vi "Three part live.vi"() -> ()   [LabVIEW 2009]
uses:
  <vilib>/vision/Image Controls.llb/IMAQ Image.ctl
  <vilib>/Instr/_visa.llb/VISA Configure Serial Port (Instr).vi
  <vilib>/userDefined/High Color/IMAQdx.ctl
  <vilib>/Analysis/3filter.llb/Filter Passband Type.ctl
  <vilib>/Analysis/3filter.llb/Butterworth Filter (DBL).vi
  <vilib>/vision/NI_Vision_Development_Module.lvlib
  <vilib>/Analysis/NI_AALBase.lvlib
  <vilib>/vision/driver/NI_Vision_Acquisition_Software.lvlib
panel:
  in  "Orange Guitar":T1={"Global Rectangle"=[587, 282, 628, 378], "Contours"=[{"ID"=enum."External", "Type"=2, "Coordinates"=[627, 377, 587, 282]}]} {"Contours"."Type" items=["No Selection", "Point", "Line", "Rectangle", "Oval", "Polygon", "Freehand Region", "Annulus", "Unused2", "Unused3", "Broken Line", "Freehand Line", "Rotated Rectangle"]}
  in  "Yellow Guitar":T1={"Global Rectangle"=[546, 282, 563, 376], "Contours"=[{"ID"=enum."External", "Type"=2, "Coordinates"=[562, 375, 546, 282]}]} {"Contours"."Type" items=["No Selection", "Point", "Line", "Rectangle", "Oval", "Polygon", "Freehand Region", "Annulus", "Unused2", "Unused3", "Broken Line", "Freehand Line", "Rotated Rectangle"]}
  in  "Green Guitar":T1={"Global Rectangle"=[498, 284, 505, 376], "Contours"=[{"ID"=enum."External", "Type"=2, "Coordinates"=[498, 375, 504, 284]}]} {"Contours"."Type" items=["No Selection", "Point", "Line", "Rectangle", "Oval", "Polygon", "Freehand Region", "Annulus", "Unused2", "Unused3", "Broken Line", "Freehand Line", "Rotated Rectangle"]}
  in  "Blue Guitar":T1={"Global Rectangle"=[569, 290, 594, 372], "Contours"=[{"ID"=enum."External", "Type"=2, "Coordinates"=[593, 371, 569, 290]}]} {"Contours"."Type" items=["No Selection", "Point", "Line", "Rectangle", "Oval", "Polygon", "Freehand Region", "Annulus", "Unused2", "Unused3", "Broken Line", "Freehand Line", "Rotated Rectangle"]}
  in  "Red Guitar":T1={"Global Rectangle"=[526, 284, 530, 370], "Contours"=[{"ID"=enum."External", "Type"=2, "Coordinates"=[529, 369, 526, 284]}]} {"Contours"."Type" items=["No Selection", "Point", "Line", "Rectangle", "Oval", "Polygon", "Freehand Region", "Annulus", "Unused2", "Unused3", "Broken Line", "Freehand Line", "Rotated Rectangle"]}
  in  "sampling  9":dbl=1.0 format="%0.2f"
  in  "high 14":dbl=60.0 format="%0.2f"
  out "Blue Guitar":dbl[](graph)
  in  "low 3":dbl=0.12500000000000006 format="%0.4f"
  out "Yellow Guitar":dbl[](graph)
  out "Yellow Guitar LED":bool
  in  "sampling 12":dbl=1.0 format="%0.2f"
  in  "high 13":dbl=60.0 format="%0.2f"
  in  "low  12":dbl=0.12500000000000006 format="%0.4f"
  out "Yellow Guitar":T1={"Global Rectangle"=[243, 262, 261, 384], "Contours"=[{"ID"=enum."External", "Type"=2, "Coordinates"=[260, 383, 243, 262]}]} {"Contours"."Type" items=["No Selection", "Point", "Line", "Rectangle", "Oval", "Polygon", "Freehand Region", "Annulus", "Unused2", "Unused3", "Broken Line", "Freehand Line", "Rotated Rectangle"]}
  out "Blue Guitar":T1={"Global Rectangle"=[168, 264, 180, 378], "Contours"=[{"ID"=enum."External", "Type"=2, "Coordinates"=[168, 377, 179, 264]}]} {"Contours"."Type" items=["No Selection", "Point", "Line", "Rectangle", "Oval", "Polygon", "Freehand Region", "Annulus", "Unused2", "Unused3", "Broken Line", "Freehand Line", "Rotated Rectangle"]}
  out "Green Guitar":dbl[](graph)
  out "Green Guitar LED":bool
  in  "sampling 11":dbl=1.0 format="%0.2f"
  in  "high 12":dbl=60.0 format="%0.2f"
  in  "low  11":dbl=0.12500000000000006 format="%0.4f"
  out "Green Guitar":T1={"Global Rectangle"=[406, 309, 423, 383], "Contours"=[{"ID"=enum."External", "Type"=2, "Coordinates"=[422, 382, 406, 309]}]} {"Contours"."Type" items=["No Selection", "Point", "Line", "Rectangle", "Oval", "Polygon", "Freehand Region", "Annulus", "Unused2", "Unused3", "Broken Line", "Freehand Line", "Rotated Rectangle"]}
  out "Red Guitar":dbl[](graph)
  out "Red Guitar LED":bool
  in  "sampling 10":dbl=1.0 format="%0.2f"
  in  "high 11":dbl=60.0 format="%0.2f"
  in  "low  10":dbl=0.12500000000000006 format="%0.4f"
  out "Red Guitar":T1={"Global Rectangle"=[300, 297, 320, 380], "Contours"=[{"ID"=enum."External", "Type"=2, "Coordinates"=[300, 379, 319, 297]}]} {"Contours"."Type" items=["No Selection", "Point", "Line", "Rectangle", "Oval", "Polygon", "Freehand Region", "Annulus", "Unused2", "Unused3", "Broken Line", "Freehand Line", "Rotated Rectangle"]}
  out "Blue Guitar LED":bool
  out "Orange Guitar":dbl[](graph)
  out "Orange Guitar LED":bool
  in  "sampling 9":dbl=1.0 format="%0.2f"
  in  "high 10":dbl=60.0 format="%0.2f"
  in  "low  9":dbl=0.12500000000000006 format="%0.4f"
  out "Orange Guitar":T1={"Global Rectangle"=[300, 297, 320, 380], "Contours"=[{"ID"=enum."External", "Type"=2, "Coordinates"=[300, 379, 319, 297]}]} {"Contours"."Type" items=["No Selection", "Point", "Line", "Rectangle", "Oval", "Polygon", "Freehand Region", "Annulus", "Unused2", "Unused3", "Broken Line", "Freehand Line", "Rotated Rectangle"]}
  in  "Orange Bass":T1={"Global Rectangle"=[220, 296, 225, 371], "Contours"=[{"ID"=enum."External", "Type"=2, "Coordinates"=[224, 370, 220, 296]}]} {"Contours"."Type" items=["No Selection", "Point", "Line", "Rectangle", "Oval", "Polygon", "Freehand Region", "Annulus", "Unused2", "Unused3", "Broken Line", "Freehand Line", "Rotated Rectangle"]}
  out "Orange Bass":dbl[](graph)
  out "Orange Bass LED":bool
  in  "sampling 8":dbl=1.0 format="%0.2f"
  in  "high 9":dbl=60.0 format="%0.2f"
  in  "low  8":dbl=0.12500000000000006 format="%0.4f"
  out "Orange Bass":T1={"Global Rectangle"=[300, 297, 320, 380], "Contours"=[{"ID"=enum."External", "Type"=2, "Coordinates"=[300, 379, 319, 297]}]} {"Contours"."Type" items=["No Selection", "Point", "Line", "Rectangle", "Oval", "Polygon", "Freehand Region", "Annulus", "Unused2", "Unused3", "Broken Line", "Freehand Line", "Rotated Rectangle"]}
  in  "Green Bass":T1={"Global Rectangle"=[100, 292, 131, 371], "Contours"=[{"ID"=enum."External", "Type"=2, "Coordinates"=[100, 370, 130, 292]}]} {"Contours"."Type" items=["No Selection", "Point", "Line", "Rectangle", "Oval", "Polygon", "Freehand Region", "Annulus", "Unused2", "Unused3", "Broken Line", "Freehand Line", "Rotated Rectangle"]}
  in  "Blue Bass":T1={"Global Rectangle"=[193, 293, 199, 374], "Contours"=[{"ID"=enum."External", "Type"=2, "Coordinates"=[193, 373, 198, 293]}]} {"Contours"."Type" items=["No Selection", "Point", "Line", "Rectangle", "Oval", "Polygon", "Freehand Region", "Annulus", "Unused2", "Unused3", "Broken Line", "Freehand Line", "Rotated Rectangle"]}
  in  "Red Bass":T1={"Global Rectangle"=[129, 294, 154, 376], "Contours"=[{"ID"=enum."External", "Type"=2, "Coordinates"=[129, 375, 153, 294]}]} {"Contours"."Type" items=["No Selection", "Point", "Line", "Rectangle", "Oval", "Polygon", "Freehand Region", "Annulus", "Unused2", "Unused3", "Broken Line", "Freehand Line", "Rotated Rectangle"]}
  in  "Yellow Bass":T1={"Global Rectangle"=[160, 295, 175, 378], "Contours"=[{"ID"=enum."External", "Type"=2, "Coordinates"=[160, 377, 174, 295]}]} {"Contours"."Type" items=["No Selection", "Point", "Line", "Rectangle", "Oval", "Polygon", "Freehand Region", "Annulus", "Unused2", "Unused3", "Broken Line", "Freehand Line", "Rotated Rectangle"]}
  in  "sampling  8":dbl=1.0 format="%0.2f"
  in  "high 8":dbl=60.0 format="%0.2f"
  out "Blue Bass":dbl[](graph)
  in  "low 2":dbl=0.12500000000000006 format="%0.4f"
  out "Yellow Bass":dbl[](graph)
  out "Yellow Bass LED":bool
  in  "sampling 7":dbl=1.0 format="%0.2f"
  in  "high 7":dbl=60.0 format="%0.2f"
  in  "low  7":dbl=0.12500000000000006 format="%0.4f"
  out "Yellow Bass":T1={"Global Rectangle"=[243, 262, 261, 384], "Contours"=[{"ID"=enum."External", "Type"=2, "Coordinates"=[260, 383, 243, 262]}]} {"Contours"."Type" items=["No Selection", "Point", "Line", "Rectangle", "Oval", "Polygon", "Freehand Region", "Annulus", "Unused2", "Unused3", "Broken Line", "Freehand Line", "Rotated Rectangle"]}
  out "Blue Bass":T1={"Global Rectangle"=[168, 264, 180, 378], "Contours"=[{"ID"=enum."External", "Type"=2, "Coordinates"=[168, 377, 179, 264]}]} {"Contours"."Type" items=["No Selection", "Point", "Line", "Rectangle", "Oval", "Polygon", "Freehand Region", "Annulus", "Unused2", "Unused3", "Broken Line", "Freehand Line", "Rotated Rectangle"]}
  out "Green Bass":dbl[](graph)
  out "Green Bass LED":bool
  in  "sampling 6":dbl=1.0 format="%0.2f"
  in  "high 6":dbl=60.0 format="%0.2f"
  in  "low  6":dbl=0.12500000000000006 format="%0.4f"
  out "Green Bass":T1={"Global Rectangle"=[406, 309, 423, 383], "Contours"=[{"ID"=enum."External", "Type"=2, "Coordinates"=[422, 382, 406, 309]}]} {"Contours"."Type" items=["No Selection", "Point", "Line", "Rectangle", "Oval", "Polygon", "Freehand Region", "Annulus", "Unused2", "Unused3", "Broken Line", "Freehand Line", "Rotated Rectangle"]}
  out "Red Bass":dbl[](graph)
  out "Red Bass LED":bool
  in  "sampling 5":dbl=1.0 format="%0.2f"
  in  "high 5":dbl=60.0 format="%0.2f"
  in  "low  5":dbl=0.12500000000000006 format="%0.4f"
  out "Red Bass":T1={"Global Rectangle"=[300, 297, 320, 380], "Contours"=[{"ID"=enum."External", "Type"=2, "Coordinates"=[300, 379, 319, 297]}]} {"Contours"."Type" items=["No Selection", "Point", "Line", "Rectangle", "Oval", "Polygon", "Freehand Region", "Annulus", "Unused2", "Unused3", "Broken Line", "Freehand Line", "Rotated Rectangle"]}
  out "Blue Bass LED":bool
  in  "Mask":T1 {"Contours"."Type" items=["No Selection", "Point", "Line", "Rectangle", "Oval", "Polygon", "Freehand Region", "Annulus", "Unused2", "Unused3", "Broken Line", "Freehand Line", "Rotated Rectangle"]}
  out "Image 2":T2(plugin-control)
  out "Red Line":T1={"Global Rectangle"=[300, 297, 320, 380], "Contours"=[{"ID"=enum."External", "Type"=2, "Coordinates"=[300, 379, 319, 297]}]} {"Contours"."Type" items=["No Selection", "Point", "Line", "Rectangle", "Oval", "Polygon", "Freehand Region", "Annulus", "Unused2", "Unused3", "Broken Line", "Freehand Line", "Rotated Rectangle"]}
  in  "Red Line":T1={"Global Rectangle"=[300, 297, 320, 380], "Contours"=[{"ID"=enum."External", "Type"=2, "Coordinates"=[300, 379, 319, 297]}]} {"Contours"."Type" items=["No Selection", "Point", "Line", "Rectangle", "Oval", "Polygon", "Freehand Region", "Annulus", "Unused2", "Unused3", "Broken Line", "Freehand Line", "Rotated Rectangle"]}
  out "Waveform Red":dbl[](graph)
  out "LED Red":bool
  in  "sampling 4":dbl=1.0 format="%0.2f"
  in  "high 4":dbl=60.0 format="%0.2f"
  in  "low  4":dbl=0.12500000000000006 format="%0.4f"
  out "Green Line":T1={"Global Rectangle"=[406, 309, 423, 383], "Contours"=[{"ID"=enum."External", "Type"=2, "Coordinates"=[422, 382, 406, 309]}]} {"Contours"."Type" items=["No Selection", "Point", "Line", "Rectangle", "Oval", "Polygon", "Freehand Region", "Annulus", "Unused2", "Unused3", "Broken Line", "Freehand Line", "Rotated Rectangle"]}
  in  "Blue Line":T1={"Global Rectangle"=[374, 278, 383, 377], "Contours"=[{"ID"=enum."External", "Type"=2, "Coordinates"=[382, 376, 374, 278]}]} {"Contours"."Type" items=["No Selection", "Point", "Line", "Rectangle", "Oval", "Polygon", "Freehand Region", "Annulus", "Unused2", "Unused3", "Broken Line", "Freehand Line", "Rotated Rectangle"]}
  in  "Green Line":T1={"Global Rectangle"=[406, 309, 423, 383], "Contours"=[{"ID"=enum."External", "Type"=2, "Coordinates"=[422, 382, 406, 309]}]} {"Contours"."Type" items=["No Selection", "Point", "Line", "Rectangle", "Oval", "Polygon", "Freehand Region", "Annulus", "Unused2", "Unused3", "Broken Line", "Freehand Line", "Rotated Rectangle"]}
  in  "low  3":dbl=0.12500000000000006 format="%0.4f"
  out "Waveform Green":dbl[](graph)
  out "LED Green":bool
  in  "sampling 3":dbl=1.0 format="%0.2f"
  in  "high 3":dbl=60.0 format="%0.2f"
  in  "Yellow Line":T1={"Global Rectangle"=[342, 292, 349, 377], "Contours"=[{"ID"=enum."External", "Type"=2, "Coordinates"=[342, 376, 348, 292]}]} {"Contours"."Type" items=["No Selection", "Point", "Line", "Rectangle", "Oval", "Polygon", "Freehand Region", "Annulus", "Unused2", "Unused3", "Broken Line", "Freehand Line", "Rotated Rectangle"]}
  out "Blue Line":T1={"Global Rectangle"=[168, 264, 180, 378], "Contours"=[{"ID"=enum."External", "Type"=2, "Coordinates"=[168, 377, 179, 264]}]} {"Contours"."Type" items=["No Selection", "Point", "Line", "Rectangle", "Oval", "Polygon", "Freehand Region", "Annulus", "Unused2", "Unused3", "Broken Line", "Freehand Line", "Rotated Rectangle"]}
  out "cluster":T3
  in  "baud rate (9600)":u32=9600
  in  "VISA resource name":refnum<visa-resource-name>
  out "number":u32
  out "decimal integer string":string
  out "Image Dst Out":T2
  out "Yellow Line":T1={"Global Rectangle"=[243, 262, 261, 384], "Contours"=[{"ID"=enum."External", "Type"=2, "Coordinates"=[260, 383, 243, 262]}]} {"Contours"."Type" items=["No Selection", "Point", "Line", "Rectangle", "Oval", "Polygon", "Freehand Region", "Annulus", "Unused2", "Unused3", "Broken Line", "Freehand Line", "Rotated Rectangle"]}
  in  "low  2":dbl=0.12500000000000006 format="%0.4f"
  in  "high 2":dbl=60.0 format="%0.2f"
  in  "sampling 2":dbl=1.0 format="%0.2f"
  out "LED Yellow":bool
  out "Waveform Yellow":dbl[](graph)
  in  "playtime":dbl=30.0
  out "Frame Number":i32
  in  "Frame Start":i32=2400
  out "Blue Drum":bool
  in  "low":dbl=0.12500000000000006 format="%0.4f"
  out "Blue Drum":dbl[](graph)
  in  "high":dbl=60.0 format="%0.2f"
  in  "sampling":dbl=1.0 format="%0.2f"
  in  "stop":bool
  # "BLUE"
  # "YELLOW"
  # "GREEN"
  # "RED"
  # "Drums"
  # "Bass"
  # "Guitar"
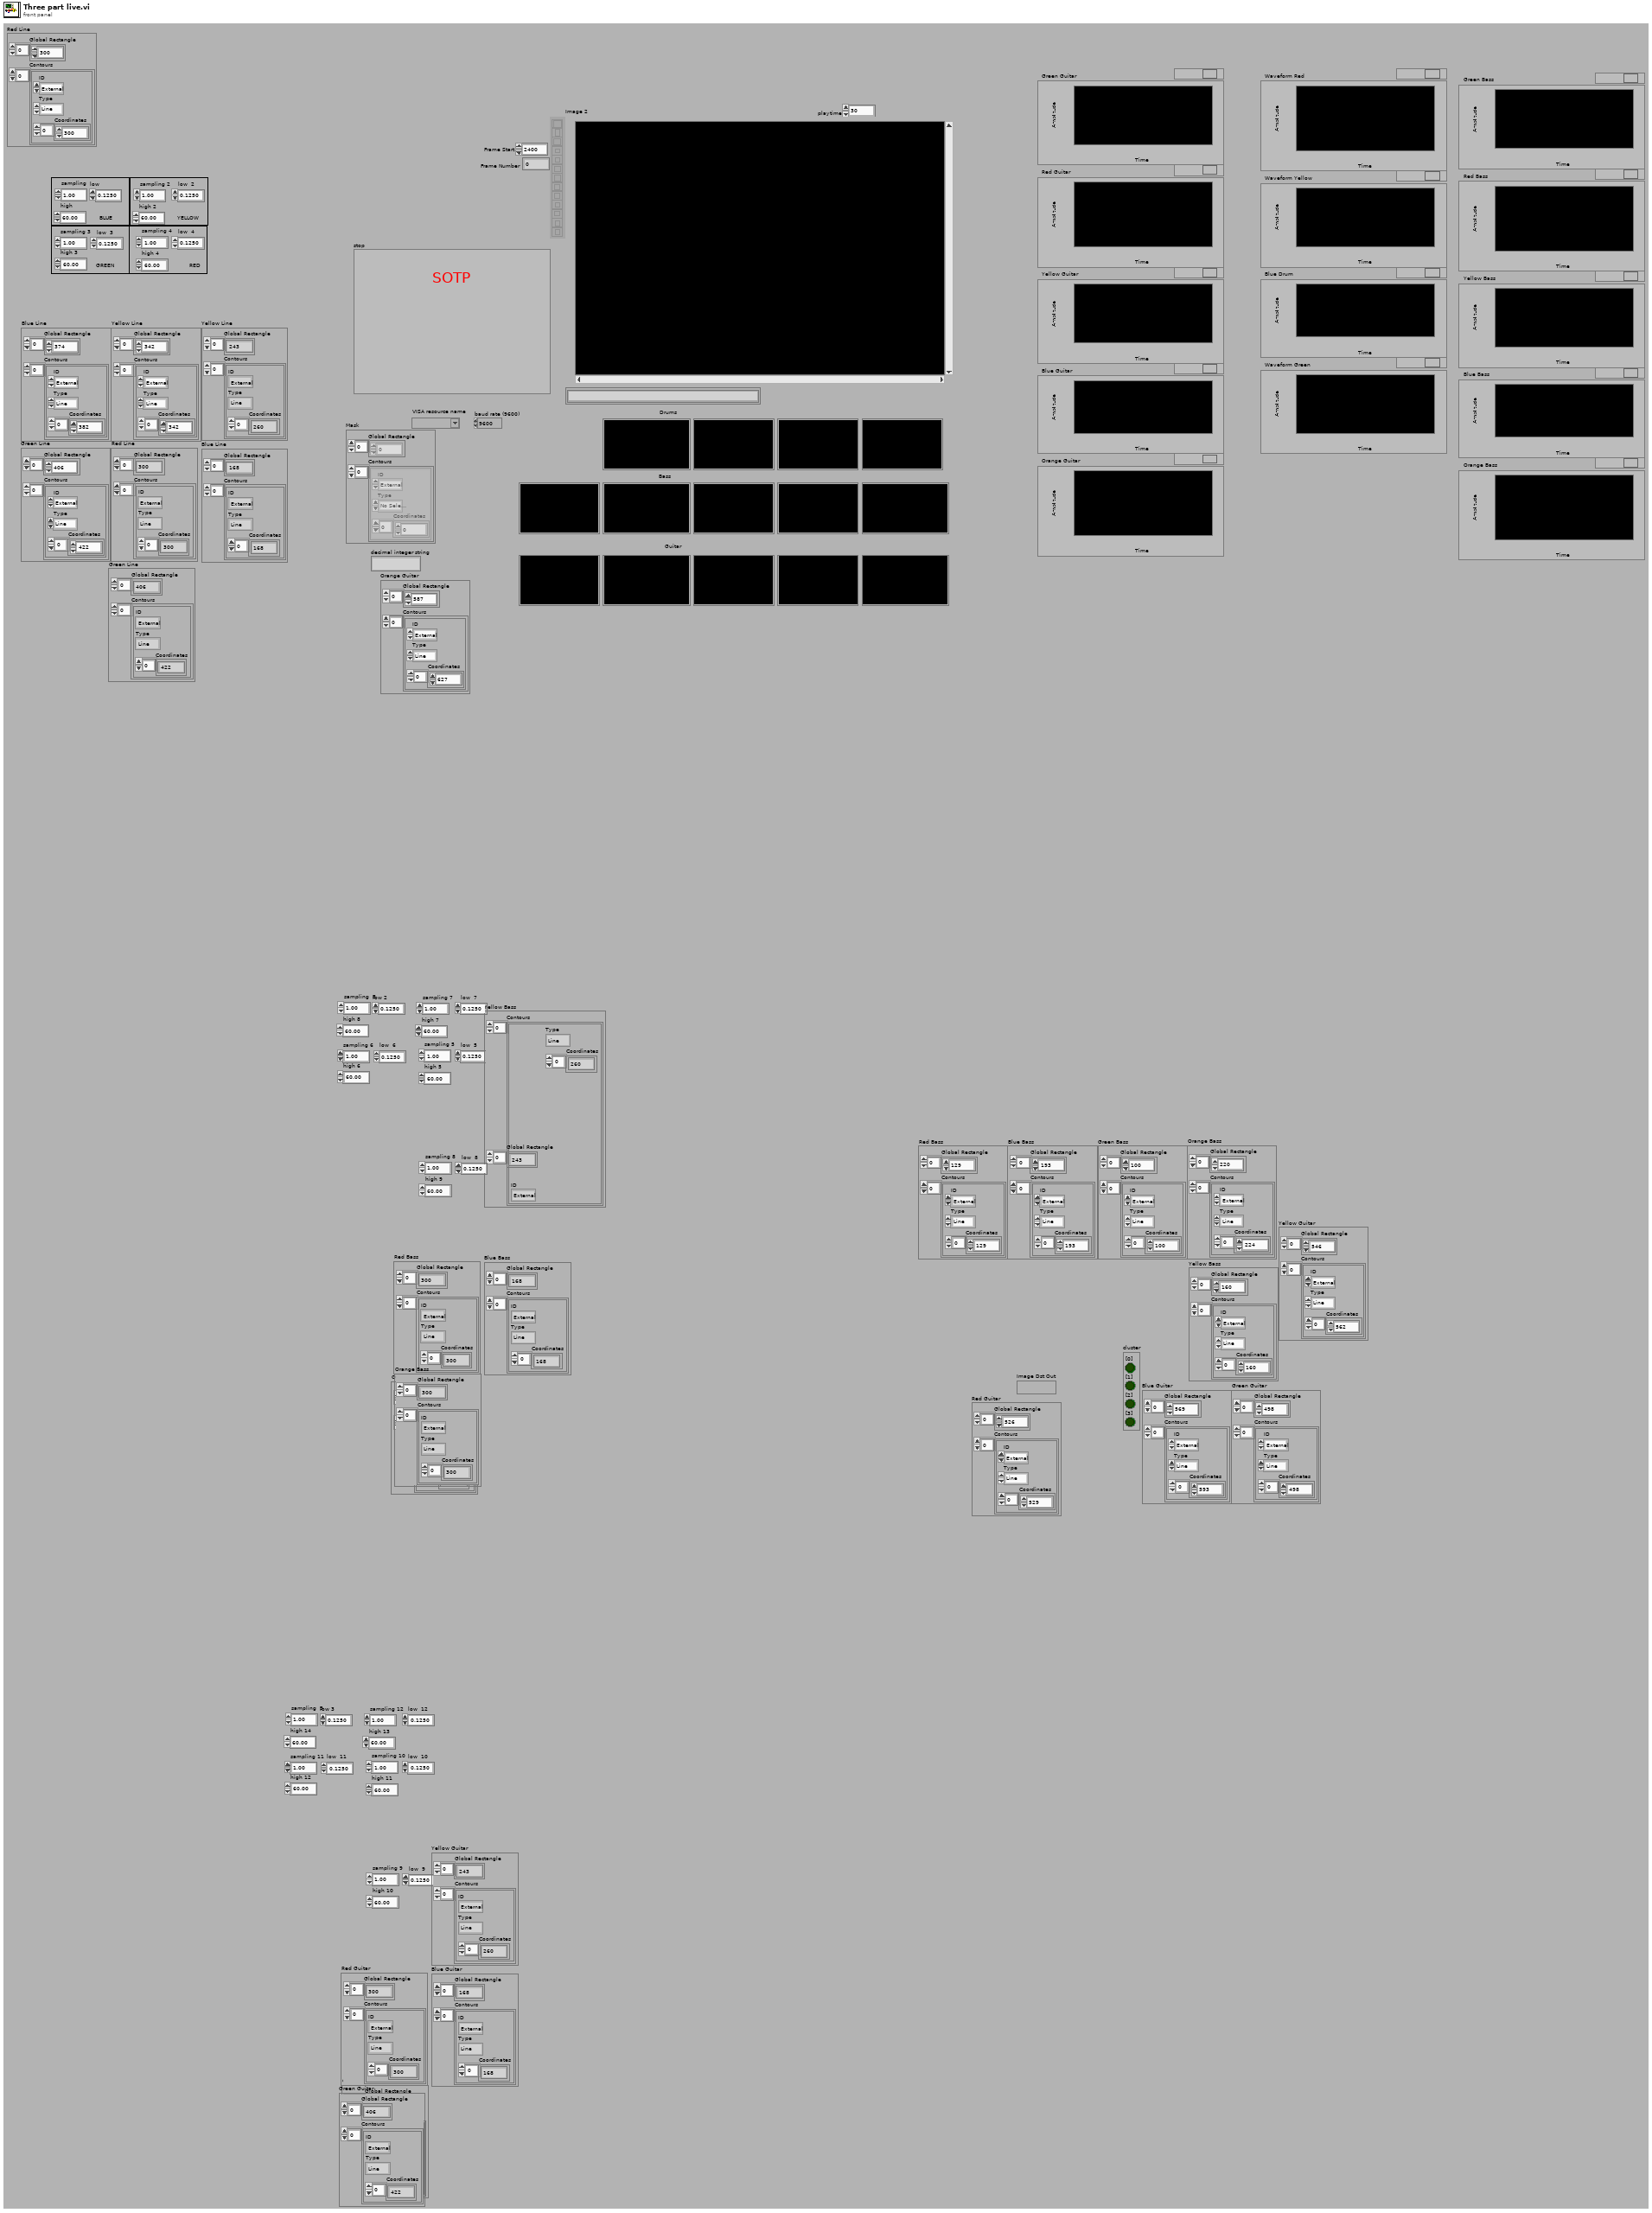
[diagram p1: front panel]
types:
  T1 = cluster{"Global Rectangle":i32[], "Contours":cluster{"ID":enum32{"External", "Internal"}, "Type":u32, "Coordinates":i32[]}[]}
  T2 = typedef "IMAQ Image.ctl" = refnum<image>
  T3 = cluster{"[0]":bool, "[1]":bool, "[2]":bool, "[3]":bool, "[4]":bool, "[5]":bool, "[6]":bool, "[7]":bool, "[8]":bool}
  T4 = typedef "IMAQdx.ctl" = refnum<k21>
  T5 = typedef "NI_AALBase.lvlib/Filter Passband Type.ctl" = enum32{"Lowpass", "Highpass", "Bandpass", "Bandstop"}
  T6 = typedef "Image Type" = u32
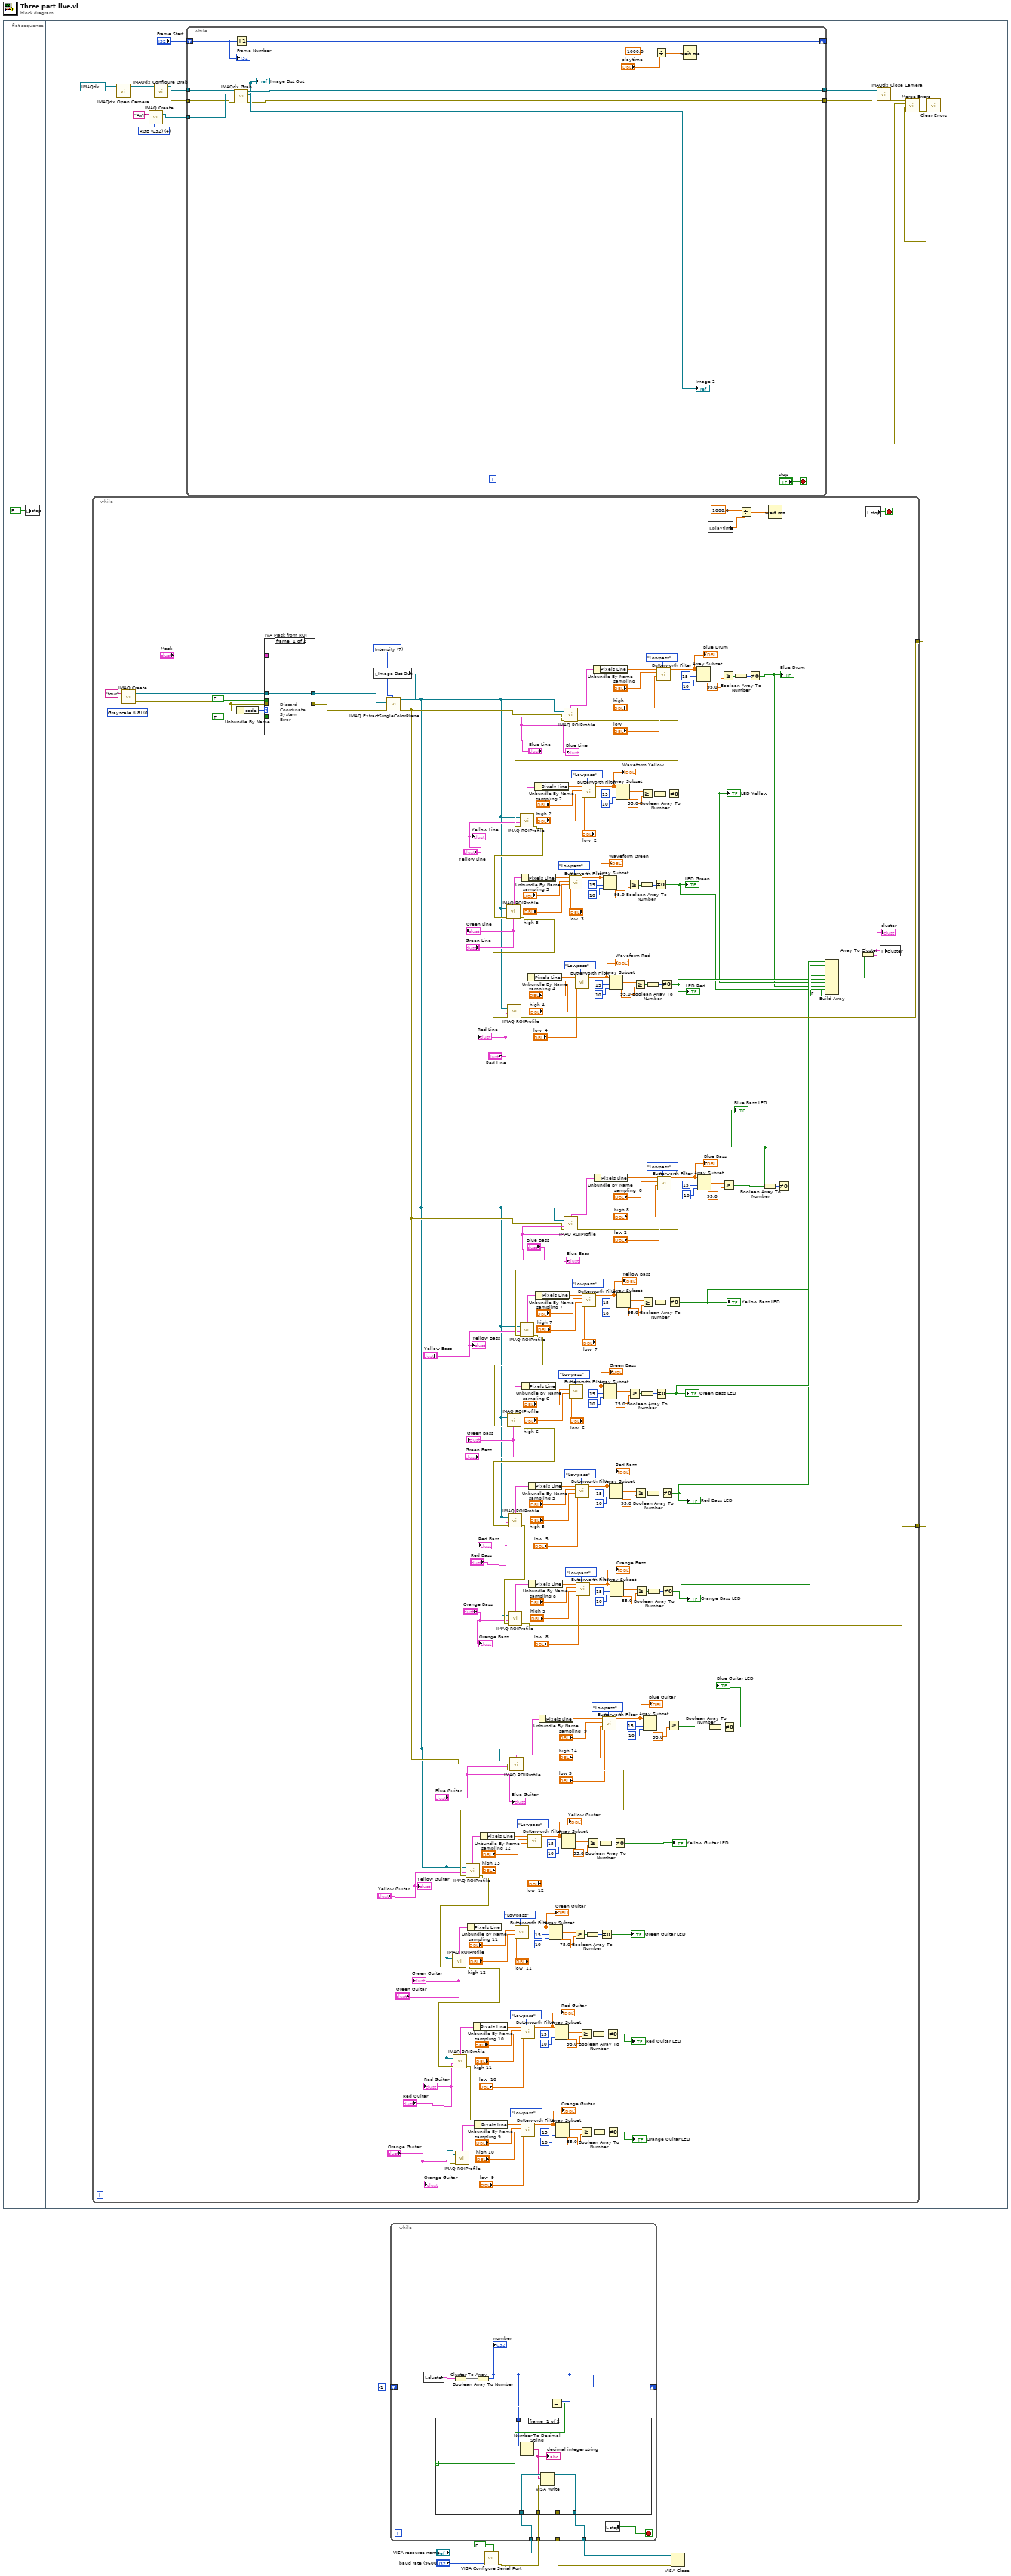
[diagram p0: block diagram]
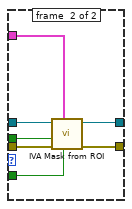
[diagram p3: hidden frame]
diagram:
  n1 = flat-sequence {
    frame #0 {
      n2 = local write "stop"(FALSE ("stop")) -> ()
    }
    frame #1 {
      w16 = T6 4 items=["Grayscale (U8)", "Grayscale (I16)", "Grayscale (SGL)", "Complex (CSG)", "RGB (U32)", "HSL (U32)", "RGB (U64)", "Grayscale (U16)"] ("Image Type")
      n3 = while {
        tunnel: [w252] -> w22
        tunnel: [w118] -> w21
        stop <- w267 stop-if-true
        w262 = T6 0 items=["Grayscale (U8)", "Grayscale (I16)", "Grayscale (SGL)", "Complex (CSG)", "RGB (U32)", "HSL (U32)", "RGB (U64)", "Grayscale (U16)"] ("Image Type")
        w268 = 7 items=["Red", "Green", "Blue", "Hue", "Saturation", "Luminance", "Value", "Intensity"] ("Color Plane")
        n4 = call "IMAQ Create"("Image Name"="four", "Image Type"=w262) -> ("New Image"=w255:T2, "error out"=w256:errorcluster)  [unwired: 3 in]
        n5 = Unbundle By Name(w256) -> ("code"=w260:i32)
        n6 = case "IVA Mask from ROI" shown="Default" w260 {
          tunnel: "Mask" -> [_ w276]
          tunnel: TRUE ("Shrink") -> [_ w275]
          tunnel: w255 -> [w269 w274]
          tunnel: w256 -> [_ w273]
          tunnel: [_ w272] -> w257
          tunnel: [w269 w271] -> w253
          tunnel: FALSE ("Out / In") -> [_ w270]
          frame #0 {
            # "Discard\nCoordinate\nSystem\nError"
          }
          frame #1 {
            n7 = call <vilib>:"IVA Mask from ROI.vi"("Shrink"=w275, "ROI Descriptor"=w276, "error in (no error)"=w273, "Out / In"=w270, "Image Src"=w274) -> ("error out"=w272:errorcluster, "Image Out"=w271:T2)  [unwired: 5 out]
          }
        }
        n8 = local read "Image Dst Out"() -> (w263:T2)
        n9 = call "IMAQ ExtractSingleColorPlane"("Color Plane"=w268, "error in (no error)"=w257, "Image Dst"=w253, "Image Src"=w263) -> ("error out"=w33:errorcluster, "Image Dst Out"=w28:T2)  [unwired: 6 out]
        n10 = call "IMAQ ROIProfile"("error in (no error)"=w33, "ROI Descriptor"="Blue Guitar", "Image"=w28) -> ("error out"=w58:errorcluster, "ROI Graph"=w59:cluster{"x0":sgl, "dx":sgl, "Pixels Line":sgl[]})  [unwired: 4 out]
        n11 = call "IMAQ ROIProfile"("error in (no error)"=w58, "ROI Descriptor"="Yellow Guitar", "Image"=w28) -> ("error out"=w88:errorcluster, "ROI Graph"=w55:cluster{"x0":sgl, "dx":sgl, "Pixels Line":sgl[]})  [unwired: 4 out]
        n12 = call "IMAQ ROIProfile"("error in (no error)"=w88, "ROI Descriptor"="Green Guitar", "Image"=w28) -> ("error out"=w87:errorcluster, "ROI Graph"=w61:cluster{"x0":sgl, "dx":sgl, "Pixels Line":sgl[]})  [unwired: 4 out]
        n13 = call "IMAQ ROIProfile"("error in (no error)"=w87, "ROI Descriptor"="Red Guitar", "Image"=w28) -> ("error out"=w27:errorcluster, "ROI Graph"=w85:cluster{"x0":sgl, "dx":sgl, "Pixels Line":sgl[]})  [unwired: 4 out]
        n14 = call "IMAQ ROIProfile"("error in (no error)"=w27, "ROI Descriptor"="Orange Guitar", "Image"=w28) -> ("ROI Graph"=w26:cluster{"x0":sgl, "dx":sgl, "Pixels Line":sgl[]})  [unwired: 5 out]
        n15 = Unbundle By Name(w61) -> ("Pixels Line"=w64:sgl[])
        n16 = Unbundle By Name(w85) -> ("Pixels Line"=w82:sgl[])
        n17 = Unbundle By Name(w26) -> ("Pixels Line"=w92:sgl[])
        n18 = Unbundle By Name(w55) -> ("Pixels Line"=w52:sgl[])
        n19 = call-poly <vilib>:"Butterworth Filter.vi"("filter type"=Filter_Passband_Type."Lowpass", "low cutoff freq: fl"="low  11", "high cutoff freq: fh"="high 12", "sampling freq: fs"="sampling 11", "X"=w64) -> ("Filtered X"=w60:dbl[])  [unwired: 3 in, 1 out]
        "Green Guitar" <- w60
        n20 = call-poly <vilib>:"Butterworth Filter.vi"("filter type"=Filter_Passband_Type."Lowpass", "low cutoff freq: fl"="low  10", "high cutoff freq: fh"="high 11", "sampling freq: fs"="sampling 10", "X"=w82) -> ("Filtered X"=w86:dbl[])  [unwired: 3 in, 1 out]
        "Red Guitar" <- w86
        n21 = call-poly <vilib>:"Butterworth Filter.vi"("filter type"=Filter_Passband_Type."Lowpass", "low cutoff freq: fl"="low  9", "high cutoff freq: fh"="high 10", "sampling freq: fs"="sampling 9", "X"=w92) -> ("Filtered X"=w89:dbl[])  [unwired: 3 in, 1 out]
        "Orange Guitar" <- w89
        n22 = call-poly <vilib>:"Butterworth Filter.vi"("filter type"=Filter_Passband_Type."Lowpass", "low cutoff freq: fl"="low  12", "high cutoff freq: fh"="high 13", "sampling freq: fs"="sampling 12", "X"=w52) -> ("Filtered X"=w56:dbl[])  [unwired: 3 in, 1 out]
        "Yellow Guitar" <- w56
        n23 = Unbundle By Name(w59) -> ("Pixels Line"=w36:sgl[])
        n24 = Array Subset(array=w60, index=15, length=10) -> (w69:dbl[])
        n25 = Array Subset(array=w86, index=15, length=10) -> (w77:dbl[])
        n26 = Array Subset(array=w89, index=15, length=10) -> (w97:dbl[])
        n27 = Array Subset(array=w56, index=15, length=10) -> (w47:dbl[])
        n28 = call "IMAQ ROIProfile"("error in (no error)"=w33, "ROI Descriptor"="Blue Line", "Image"=w28) -> ("error out"=w227:errorcluster, "ROI Graph"=w226:cluster{"x0":sgl, "dx":sgl, "Pixels Line":sgl[]})  [unwired: 4 out]
        n29 = call "IMAQ ROIProfile"("error in (no error)"=w227, "ROI Descriptor"="Yellow Line", "Image"=w28) -> ("error out"=w194:errorcluster, "ROI Graph"=w230:cluster{"x0":sgl, "dx":sgl, "Pixels Line":sgl[]})  [unwired: 4 out]
        n30 = call "IMAQ ROIProfile"("error in (no error)"=w194, "ROI Descriptor"="Green Line", "Image"=w28) -> ("error out"=w197:errorcluster, "ROI Graph"=w224:cluster{"x0":sgl, "dx":sgl, "Pixels Line":sgl[]})  [unwired: 4 out]
        n31 = call "IMAQ ROIProfile"("error in (no error)"=w197, "ROI Descriptor"="Red Line", "Image"=w28) -> ("error out"=w252:errorcluster, "ROI Graph"=w199:cluster{"x0":sgl, "dx":sgl, "Pixels Line":sgl[]})  [unwired: 4 out]
        n32 = Unbundle By Name(w224) -> ("Pixels Line"=w221:sgl[])
        n33 = Unbundle By Name(w199) -> ("Pixels Line"=w202:sgl[])
        n34 = Unbundle By Name(w230) -> ("Pixels Line"=w233:sgl[])
        n35 = call "IMAQ ROIProfile"("error in (no error)"=w33, "ROI Descriptor"="Blue Bass", "Image"=w28) -> ("error out"=w167:errorcluster, "ROI Graph"=w166:cluster{"x0":sgl, "dx":sgl, "Pixels Line":sgl[]})  [unwired: 4 out]
        n36 = call "IMAQ ROIProfile"("error in (no error)"=w167, "ROI Descriptor"="Yellow Bass", "Image"=w28) -> ("error out"=w137:errorcluster, "ROI Graph"=w170:cluster{"x0":sgl, "dx":sgl, "Pixels Line":sgl[]})  [unwired: 4 out]
        n37 = call "IMAQ ROIProfile"("error in (no error)"=w137, "ROI Descriptor"="Green Bass", "Image"=w28) -> ("error out"=w138:errorcluster, "ROI Graph"=w164:cluster{"x0":sgl, "dx":sgl, "Pixels Line":sgl[]})  [unwired: 4 out]
        n38 = call "IMAQ ROIProfile"("error in (no error)"=w138, "ROI Descriptor"="Red Bass", "Image"=w28) -> ("error out"=w119:errorcluster, "ROI Graph"=w140:cluster{"x0":sgl, "dx":sgl, "Pixels Line":sgl[]})  [unwired: 4 out]
        n39 = call "IMAQ ROIProfile"("error in (no error)"=w119, "ROI Descriptor"="Orange Bass", "Image"=w28) -> ("error out"=w118:errorcluster, "ROI Graph"=w131:cluster{"x0":sgl, "dx":sgl, "Pixels Line":sgl[]})  [unwired: 4 out]
        n40 = Unbundle By Name(w164) -> ("Pixels Line"=w161:sgl[])
        n41 = Unbundle By Name(w140) -> ("Pixels Line"=w143:sgl[])
        n42 = Unbundle By Name(w131) -> ("Pixels Line"=w128:sgl[])
        n43 = Unbundle By Name(w170) -> ("Pixels Line"=w173:sgl[])
        n44 = call-poly <vilib>:"Butterworth Filter.vi"("filter type"=Filter_Passband_Type."Lowpass", "low cutoff freq: fl"="low  3", "high cutoff freq: fh"="high 3", "sampling freq: fs"="sampling 3", "X"=w221) -> ("Filtered X"=w225:dbl[])  [unwired: 3 in, 1 out]
        "Waveform Green" <- w225
        n45 = call-poly <vilib>:"Butterworth Filter.vi"("filter type"=Filter_Passband_Type."Lowpass", "low cutoff freq: fl"="low  6", "high cutoff freq: fh"="high 6", "sampling freq: fs"="sampling 6", "X"=w161) -> ("Filtered X"=w165:dbl[])  [unwired: 3 in, 1 out]
        "Green Bass" <- w165
        n46 = Greater Or Equal?(x=w69, y=75.0) -> (x >= y?=w67:bool[])
        n47 = call-poly <vilib>:"Butterworth Filter.vi"("filter type"=Filter_Passband_Type."Lowpass", "low cutoff freq: fl"="low  4", "high cutoff freq: fh"="high 4", "sampling freq: fs"="sampling 4", "X"=w202) -> ("Filtered X"=w198:dbl[])  [unwired: 3 in, 1 out]
        "Waveform Red" <- w198
        n48 = call-poly <vilib>:"Butterworth Filter.vi"("filter type"=Filter_Passband_Type."Lowpass", "low cutoff freq: fl"="low  5", "high cutoff freq: fh"="high 5", "sampling freq: fs"="sampling 5", "X"=w143) -> ("Filtered X"=w139:dbl[])  [unwired: 3 in, 1 out]
        "Red Bass" <- w139
        n49 = call-poly <vilib>:"Butterworth Filter.vi"("filter type"=Filter_Passband_Type."Lowpass", "low cutoff freq: fl"="low  8", "high cutoff freq: fh"="high 9", "sampling freq: fs"="sampling 8", "X"=w128) -> ("Filtered X"=w132:dbl[])  [unwired: 3 in, 1 out]
        "Orange Bass" <- w132
        n50 = Greater Or Equal?(x=w77, y=95.0) -> (x >= y?=w79:bool[])
        n51 = Greater Or Equal?(x=w97, y=85.0) -> (x >= y?=w95:bool[])
        n52 = call-poly <vilib>:"Butterworth Filter.vi"("filter type"=Filter_Passband_Type."Lowpass", "low cutoff freq: fl"="low  2", "high cutoff freq: fh"="high 2", "sampling freq: fs"="sampling 2", "X"=w233) -> ("Filtered X"=w229:dbl[])  [unwired: 3 in, 1 out]
        "Waveform Yellow" <- w229
        n53 = call-poly <vilib>:"Butterworth Filter.vi"("filter type"=Filter_Passband_Type."Lowpass", "low cutoff freq: fl"="low  7", "high cutoff freq: fh"="high 7", "sampling freq: fs"="sampling 7", "X"=w173) -> ("Filtered X"=w169:dbl[])  [unwired: 3 in, 1 out]
        "Yellow Bass" <- w169
        n54 = Boolean Array To Number(Boolean array=w67) -> (number=w66:u32)
        n55 = Greater Or Equal?(x=w47, y=95.0) -> (x >= y?=w49:bool[])
        n56 = Boolean Array To Number(Boolean array=w79) -> (number=w80:u32)
        n57 = Boolean Array To Number(Boolean array=w95) -> (number=w94:u32)
        n58 = Unbundle By Name(w226) -> ("Pixels Line"=w250:sgl[])
        n59 = Unbundle By Name(w166) -> ("Pixels Line"=w189:sgl[])
        n60 = Boolean Array To Number(Boolean array=w49) -> (number=w50:u32)
        n61 = Not Equal To 0?(x=w66) -> (x != 0?=→"Green Guitar LED":bool)
        n62 = call-poly <vilib>:"Butterworth Filter.vi"("filter type"=Filter_Passband_Type."Lowpass", "low cutoff freq: fl"="low 3", "high cutoff freq: fh"="high 14", "sampling freq: fs"="sampling  9", "X"=w36) -> ("Filtered X"=w73:dbl[])  [unwired: 3 in, 1 out]
        "Blue Guitar" <- w73
        n63 = Array Subset(array=w225, index=15, length=10) -> (w216:dbl[])
        n64 = Array Subset(array=w165, index=15, length=10) -> (w156:dbl[])
        n65 = Not Equal To 0?(x=w80) -> (x != 0?=→"Red Guitar LED":bool)
        n66 = Not Equal To 0?(x=w94) -> (x != 0?=→"Orange Guitar LED":bool)
        n67 = Array Subset(array=w198, index=15, length=10) -> (w207:dbl[])
        n68 = Array Subset(array=w139, index=15, length=10) -> (w148:dbl[])
        n69 = Array Subset(array=w132, index=15, length=10) -> (w123:dbl[])
        n70 = Not Equal To 0?(x=w50) -> (x != 0?=→"Yellow Guitar LED":bool)
        n71 = Array Subset(array=w229, index=15, length=10) -> (w238:dbl[])
        n72 = Array Subset(array=w169, index=15, length=10) -> (w178:dbl[])
        n73 = Greater Or Equal?(x=w216, y=95.0) -> (x >= y?=w218:bool[])
        n74 = Greater Or Equal?(x=w156, y=75.0) -> (x >= y?=w158:bool[])
        n75 = Greater Or Equal?(x=w207, y=95.0) -> (x >= y?=w205:bool[])
        n76 = Greater Or Equal?(x=w148, y=95.0) -> (x >= y?=w146:bool[])
        n77 = Greater Or Equal?(x=w123, y=85.0) -> (x >= y?=w125:bool[])
        n78 = Boolean Array To Number(Boolean array=w218) -> (number=w219:u32)
        n79 = Greater Or Equal?(x=w238, y=95.0) -> (x >= y?=w236:bool[])
        n80 = Boolean Array To Number(Boolean array=w158) -> (number=w159:u32)
        n81 = Greater Or Equal?(x=w178, y=95.0) -> (x >= y?=w176:bool[])
        n82 = Array Subset(array=w73, index=15, length=10) -> (w42:dbl[])
        n83 = Boolean Array To Number(Boolean array=w205) -> (number=w204:u32)
        n84 = Boolean Array To Number(Boolean array=w146) -> (number=w145:u32)
        n85 = Boolean Array To Number(Boolean array=w125) -> (number=w126:u32)
        n86 = Boolean Array To Number(Boolean array=w236) -> (number=w235:u32)
        n87 = Boolean Array To Number(Boolean array=w176) -> (number=w175:u32)
        n88 = Not Equal To 0?(x=w219) -> (x != 0?=w108:bool)
        "LED Green" <- w108
        n89 = Not Equal To 0?(x=w159) -> (x != 0?=w116:bool)
        "Green Bass LED" <- w116
        n90 = call-poly <vilib>:"Butterworth Filter.vi"("filter type"=Filter_Passband_Type."Lowpass", "low cutoff freq: fl"="low", "high cutoff freq: fh"="high", "sampling freq: fs"="sampling", "X"=w250) -> ("Filtered X"=w212:dbl[])  [unwired: 3 in, 1 out]
        "Blue Drum" <- w212
        n91 = call-poly <vilib>:"Butterworth Filter.vi"("filter type"=Filter_Passband_Type."Lowpass", "low cutoff freq: fl"="low 2", "high cutoff freq: fh"="high 8", "sampling freq: fs"="sampling  8", "X"=w189) -> ("Filtered X"=w152:dbl[])  [unwired: 3 in, 1 out]
        "Blue Bass" <- w152
        n92 = Not Equal To 0?(x=w204) -> (x != 0?=w111:bool)
        "LED Red" <- w111
        n93 = Not Equal To 0?(x=w145) -> (x != 0?=w115:bool)
        "Red Bass LED" <- w115
        n94 = Not Equal To 0?(x=w126) -> (x != 0?=w112:bool)
        "Orange Bass LED" <- w112
        n95 = Not Equal To 0?(x=w235) -> (x != 0?=w110:bool)
        "LED Yellow" <- w110
        n96 = Greater Or Equal?(x=w42, y=95.0) -> (x >= y?=w105:bool[])
        n97 = Not Equal To 0?(x=w175) -> (x != 0?=w114:bool)
        "Yellow Bass LED" <- w114
        n98 = Array Subset(array=w212, index=15, length=10) -> (w244:dbl[])
        n99 = Array Subset(array=w152, index=15, length=10) -> (w183:dbl[])
        n100 = local read "playtime"() -> (w264:dbl)
        n101 = Boolean Array To Number(Boolean array=w105) -> (number=w44:u32)
        n102 = Greater Or Equal?(x=w244, y=95.0) -> (x >= y?=w242:bool[])
        n103 = Greater Or Equal?(x=w183, y=95.0) -> (x >= y?=w106:bool[])
        n104 = Not Equal To 0?(x=w44) -> (x != 0?=→"Blue Guitar LED":bool)
        n105 = Boolean Array To Number(Boolean array=w242) -> (number=w241:u32)
        n106 = Divide(x=1000.0, y=w264) -> (x/y=w266:dbl)
        n107 = Not Equal To 0?(x=w241) -> (x != 0?=w109:bool)
        "Blue Drum" <- w109
        n108 = Boolean Array To Number(Boolean array=w106) -> (number=w181:u32)
        n109 = Wait (ms)(milliseconds to wait=w266) -> ()  [unwired: 1 out]
        n110 = Not Equal To 0?(x=w181) -> (x != 0?=w113:bool)
        "Blue Bass LED" <- w113
        n111 = Build Array(w116, w115, w114, w113, w112, w111, w110, w109, w108, FALSE ("element")) -> (w192:bool[])
        n112 = Array To Cluster(array=w192) -> (cluster=w193:T3)
        "cluster" <- w193
        n113 = local read "stop"() -> (w267:bool)
        n114 = local write "cluster"(w193) -> ()
        "Yellow Line" <- "Yellow Line"
        "Blue Line" <- "Blue Line"
        "Green Line" <- "Green Line"
        "Red Line" <- "Red Line"
        "Yellow Bass" <- "Yellow Bass"
        "Blue Bass" <- "Blue Bass"
        "Green Bass" <- "Green Bass"
        "Red Bass" <- "Red Bass"
        "Orange Bass" <- "Orange Bass"
        "Yellow Guitar" <- "Yellow Guitar"
        "Blue Guitar" <- "Blue Guitar"
        "Green Guitar" <- "Green Guitar"
        "Red Guitar" <- "Red Guitar"
        "Orange Guitar" <- "Orange Guitar"
      }
      n115 = call <vilib>:"IMAQdx Open Camera.vi"("Session In"=T4 "cam0") -> ("error out"=w18:errorcluster, "Session Out"=w19:T4)  [unwired: 9 in]
      n116 = call "IMAQ Create"("Image Name"="AVI", "Image Type"=w16) -> ("New Image"=w13:T2)  [unwired: 3 in, 1 out]
      n117 = call <vilib>:"IMAQdx Configure Grab.vi"("error in"=w18, "Session In"=w19) -> ("error out"=w14:errorcluster, "Session Out"=w15:T4)  [unwired: 8 in]
      n118 = while {
        tunnel: w15 -> [w282]
        tunnel: w14 -> [w280]
        tunnel: [w279] -> w12
        shift-right: [w284] -> _
        shift-left: "Frame Start" -> [w283]
        tunnel: [w277] -> w11
        tunnel: w13 -> [w281]
        stop <- "stop" stop-if-true
        n119 = call <vilib>:"IMAQdx Grab.vi"("error in"=w280, "Image In"=w281, "Session In"=w282) -> ("error out"=w277:errorcluster, "Image Out"=→"Image Dst Out" →"Image 2":T2, "Session Out"=w279:T4)  [unwired: 5 in, 1 out]
        n120 = Increment(x=w283) -> (x+1=w284:i32)
        n121 = Divide(x=1000.0, y="playtime") -> (x/y=w287:dbl)
        n122 = Wait (ms)(milliseconds to wait=w287) -> ()  [unwired: 1 out]
        "Frame Number" <- w283
      }
      n123 = call <vilib>:"IMAQdx Close Camera.vi"("error in"=w11, "Session In"=w12) -> ("error out"=w10:errorcluster)  [unwired: 9 in]
      n124 = call <vilib>:"Merge Errors.vi"("error in 3 (no error)"=w21, "error in 2 (no error)"=w22, "error in 1 (no error)"=w10) -> ("error out"=w23:errorcluster)  [unwired: 4 in]
      n125 = call <vilib>:"Clear Errors.vi"("error in (no error)"=w23) -> ()  [unwired: 6 in, 1 out]
    }
  }
  n126 = call-poly "VISA Configure Serial Port"("VISA resource name"="VISA resource name", "Enable Termination\nChar (T)"=FALSE ("Enable Termination\nChar (T)"), "baud rate (9600)"="baud rate (9600)") -> ("VISA resource name out"=w7:refnum<visa-resource-name>, "error out"=w2:errorcluster)  [unwired: 11 in]
  n127 = while {
    shift-right: [w292] -> _
    shift-left: -1 -> [w298]
    tunnel: w7 -> [w296]
    tunnel: [w295] -> w6
    tunnel: w2 -> [w294]
    tunnel: [w293] -> w1
    stop <- w289 stop-if-true
    n128 = local read "cluster"() -> (w290:T3)
    n129 = Cluster To Array(cluster=w290) -> (array=w291:bool[])
    n130 = Boolean Array To Number(Boolean array=w291) -> (number=w292:u32)
    "number" <- w292
    n131 = Equal?(x=w292, y=w298) -> (x = y?=w297:bool)
    n132 = case shown="False" w297 {
      tunnel: w296 -> [w304 w306]
      tunnel: [w303 w306] -> w295
      tunnel: w292 -> [w301 _]
      tunnel: w294 -> [w300 w305]
      tunnel: [w299 w305] -> w293
      frame #0 {
        n133 = Number To Decimal String(number=w301) -> (decimal integer string=w302:string)  [unwired: 1 in]
        "decimal integer string" <- w302
        n134 = VISA Write(VISA resource name=w304, write buffer=w302, error in (no error)=w300) -> (VISA resource name out=w303:refnum<visa-resource-name>, error out=w299:errorcluster)  [unwired: 1 out]
      }
      frame #1 {
      }
    }
    n135 = local read "stop"() -> (w289:bool)
  }
  n136 = VISA Close(VISA resource name=w6, error in (no error)=w1) -> ()  [unwired: 1 out]
